vi "Item Remove.vi"(0 "Tree Reference In":refnum<vi>, 2 "Remove Tag (Current)":string, 5 "error in (no error)":errorcluster) -> (14 "Tree Reference Out":refnum<vi>, 19 "error out":errorcluster)   [LabVIEW 2013, in "QuickVIew.lvlib"]
doc: "Deletes item from tree along with any children. Uses the current selection if there is no item input. If there is no item selected within the tree it deletes nothing. Returns error code 1136 if an invalid tag is passed in"
uses:
  QuickVIew.lvlib
panel:
  # "VI INPUTS"
  # "VI OUTPUTS"
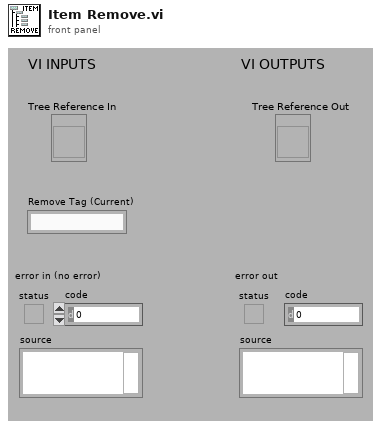
[diagram p1: front panel]
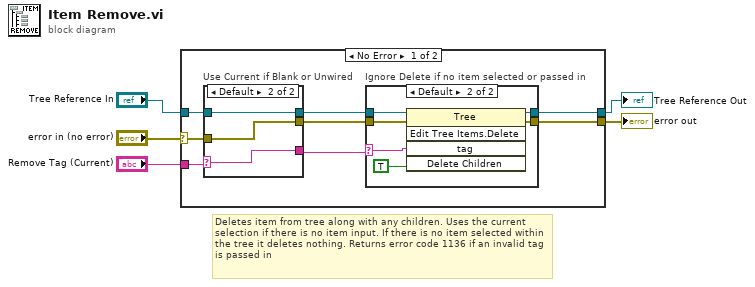
[diagram p0: block diagram]
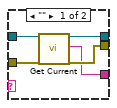
[diagram p3: hidden frame]
diagram:
  # "Deletes item from tree along with any children. Uses the current selection if there is no item input. If there is no item selected within the tree it deletes nothing. Returns error code 1136 if an invalid tag is passed in"
  n1 = case shown="No Error" "error in (no error)" {
    selector: "error in (no error)" -> [w11 w30]
    tunnel: "Tree Reference In" -> [w13 w31]
    tunnel: [w10 w31] -> w4
    tunnel: [w9 w30] -> w3
    tunnel: "Remove Tag (Current)" -> [w12 _]
    frame No Error {
      n2 = case "Use Current if Blank or Unwired" shown="Default" w12 {
        selector: w12 -> [_ w27]
        tunnel: [w25 w29] -> w8
        tunnel: w13 -> [w26 w29]
        tunnel: [w24 w28] -> w7
        tunnel: w11 -> [w23 w28]
        tunnel: [w22 w27] -> w6
        frame "" {
          n3 = call "Get Current.vi"("Tree Reference In"=w26, "error in (no error)"=w23) -> ("Tree Reference Out"=w25:refnum<vi>, "Current Tag"=w22:string, "error out"=w24:errorcluster)  [unwired: 15 out]
        }
        frame Default {
        }
      }
      n4 = case "Ignore Delete if no item selected or passed in" shown="Default" w6 {
        selector: w6 -> [_ w16]
        tunnel: [w15 w21] -> w10
        tunnel: [w14 w20] -> w9
        tunnel: w8 -> [w15 w18]
        tunnel: w7 -> [w14 w17]
        frame "" {
        }
        frame Default {
          n5 = invoke class="Tree" method="Edit Tree Items.Delete"(reference=w18, error in=w17, "tag"=w16, "Delete Children"=TRUE ("Carry Children")) -> (reference out=w21:refnum<vi>, error out=w20:errorcluster)  [unwired: 1 in, 3 out]
        }
      }
    }
    frame Error {
    }
  }
  "Tree Reference Out" <- w4
  "error out" <- w3
